vi "LINC Set Item States.vi"(4 "state values":i64[](array[numeric]), 6 "states names":string[](array[string]), 7 "item name":string, 8 "error in (no error)":errorcluster, 9 "packet name":string, 10 "type":enum16{"CMD", "TLM"}(ring), 11 "LINC session":refnum<class "LINC.lvclass">) -> (0 "error out":errorcluster, 3 "dup LINC session":refnum<class "LINC.lvclass">)   [LabVIEW 2018, in "STEPkgDriver_LINC.lvlib" / "LINC.lvclass"]
uses:
  LINC.lvclass
  LINC Global Mode.ctl
  STEPkgDriver_LINC.lvlib
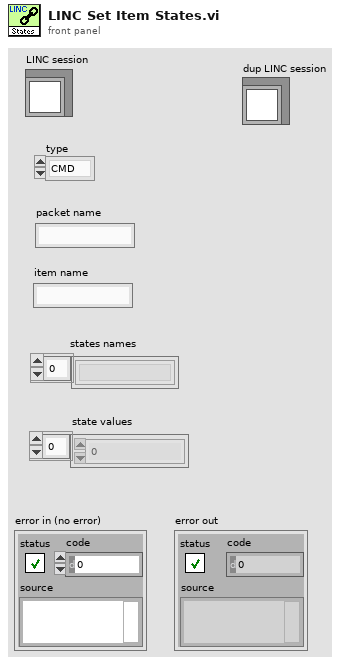
[diagram p1: front panel]
types:
  T1 = typedef "STEPkgDriver_LINC.lvlib/LINC Global Mode.ctl" = enum16{"INIT", "CLEAR", "ADD_PKT_HDR", "ADD_PKT", "GET_PKT_NAMES", "GET_PKT_DESC", "GET_PKT_HDR", "GET_PKT", "SET_PKT", "SET_DATA", "SIM_EN", "SIM_DS"}
  T2 = typedef "STEPkgDriver_LINC.lvlib/LINC Format Prototype.ctl" = cluster{"type":string, "bit offset":i32, "bit size":i32, "format":string, "unit":string, "description":string, "state values":i64[], "states":string[], "max":string, "min":string, "default":string, "array":bool, "bit element size":i32, "poly bound":dbl[], "poly scale":cluster{"coefficients":dbl[]}[], "labview size":i32, "simulate":bool, "ID":bool, "required":bool}
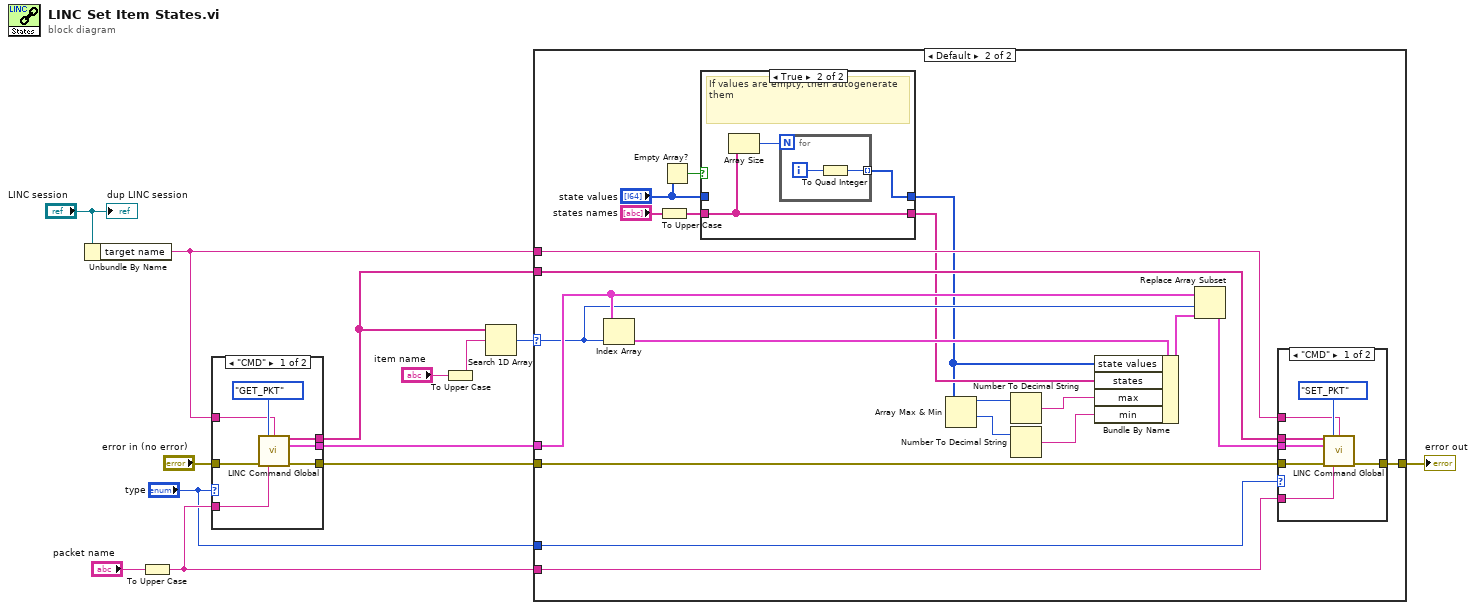
[diagram p0: block diagram]
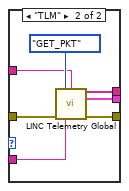
[diagram p2: hidden frame]
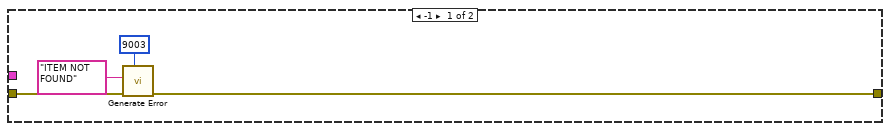
[diagram p3: hidden frame]
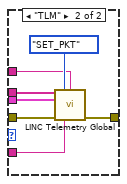
[diagram p5: hidden frame]
diagram:
  n1 = Unbundle By Name("LINC session") -> ("target name"=w3:string)
  n2 = To Upper Case(1:"packet name") -> (0:w2:string)
  n3 = case shown="\"CMD\"" "type" {
    tunnel: "error in (no error)" -> [w19 w27]
    tunnel: [w18 w25] -> w9
    tunnel: [w14 w24] -> w5
    tunnel: [w15 w23] -> w4
    tunnel: w3 -> [w17 w22]
    tunnel: w2 -> [w16 w21]
    frame "CMD" {
      n4 = call "LINC Command Global.vi"("mode"=LINC_Global_Mode."GET_PKT", "target name"=w17, "error in (no error)"=w19, "packet name"=w16) -> ("values out"=w15:string[], "item formats out"=w14:T2[], "error out"=w18:errorcluster)  [unwired: 7 in, 2 out]
    }
    frame "TLM" {
      n5 = call "LINC Telemetry Global.vi"("mode"=LINC_Global_Mode."GET_PKT", "target name"=w22, "error in (no error)"=w27, "packet name"=w21) -> ("values out"=w23:string[], "item formats out"=w24:T2[], "error out"=w25:errorcluster)  [unwired: 7 in, 2 out]
    }
  }
  n6 = To Upper Case(1:"item name") -> (0:w7:string)
  n7 = Search 1D Array(1D array=w4, element=w7) -> (index of element=w6:i32)  [unwired: 1 in]
  n8 = case shown="Default" w6 {
    selector: w6 -> [_ w48]
    tunnel: [w30 w52] -> w12
    tunnel: w9 -> [w31 w51]
    tunnel: w3 -> [_ w44]
    tunnel: w2 -> [_ w43]
    tunnel: w5 -> [_ w49]
    tunnel: w4 -> [_ w45]
    tunnel: "type" -> [_ w42]
    frame -1 {
      n9 = call "Generate Error.vi"("error code (-1301)"=9003, "error in"=w31, "description"="ITEM NOT FOUND") -> ("error out"=w30:errorcluster)  [unwired: 8 in]
    }
    frame Default {
      n10 = Index Array(array=w49, index=w48) -> (element=w50:T2)
      n11 = To Upper Case(1:"states names") -> (0:w37:string[])
      n12 = Empty Array?(array="state values") -> (empty?=w39:bool)
      n13 = case shown="True" w39 {
        tunnel: "state values" -> [w54 _]
        tunnel: [w54 w55] -> w36
        tunnel: w37 -> [w53 w57]
        tunnel: [w53 w57] -> w38
        frame False {
        }
        frame True {
          # "If values are empty, then autogenerate them"
          n14 = Array Size(array=w57) -> (size(s)=w56:i32)
          n15 = for {
            N: w56 -> [_]
            tunnel: [w58] -> w55 mode=indexing
            i -> [w59]
            n16 = To Quad Integer(1:w59) -> (0:w58:i64)
          }
        }
      }
      n17 = Array Max & Min(array=w36) -> (max value=w35:i64, min value=w33:i64)  [unwired: 2 out]
      n18 = Number To Decimal String(number=w35) -> (decimal integer string=w34:string)  [unwired: 1 in]
      n19 = Number To Decimal String(number=w33) -> (decimal integer string=w32:string)  [unwired: 1 in]
      n20 = Bundle By Name(cluster=w50, "state values"=w36, "states"=w38, "max"=w34, "min"=w32) -> (w47:T2)
      n21 = Replace Array Subset(array=w49, new element=w47, index=w48) -> (w46:T2[])
      n22 = case shown="\"CMD\"" w42 {
        tunnel: [w65 w72] -> w52
        tunnel: w51 -> [w64 w71]
        tunnel: w46 -> [w63 w70]
        tunnel: w45 -> [w62 w69]
        tunnel: w44 -> [w61 w68]
        tunnel: w43 -> [w60 w67]
        frame "CMD" {
          n23 = call "LINC Command Global.vi"("item names in"=w62, "mode"=LINC_Global_Mode."SET_PKT", "target name"=w61, "item formats in"=w63, "error in (no error)"=w64, "packet name"=w60) -> ("error out"=w65:errorcluster)  [unwired: 5 in, 4 out]
        }
        frame "TLM" {
          n24 = call "LINC Telemetry Global.vi"("item names in"=w69, "mode"=LINC_Global_Mode."SET_PKT", "target name"=w68, "item formats in"=w70, "error in (no error)"=w71, "packet name"=w67) -> ("error out"=w72:errorcluster)  [unwired: 5 in, 4 out]
        }
      }
    }
  }
  "error out" <- w12
  "dup LINC session" <- "LINC session"
